vi "PH_gentec_M-Link.Evt Call Set Auto Range.vi"(0 "i ref in":refnum<vi>, 2 "Instance":string, 3 "Set Auto Range":bool, 5 "error in (no error)":errorcluster) -> (14 "i ref out":refnum<vi>, 19 "error out":errorcluster)   [LabVIEW 2014, in "PH_gentec_M-Link.lvlib"]
doc: "This VI calls a certain Proc Event by a simple call."
uses:
  PH_gentec_M-Link.lvlib
  CS_Core/CSSystem/CoreLib/CoreLib.short 2 byte array.vi
  CS_Core/BaseProcess/BaseProcess.lvlib
  CS_Core/CSSystem/CoreLib/CoreLib.lvlib
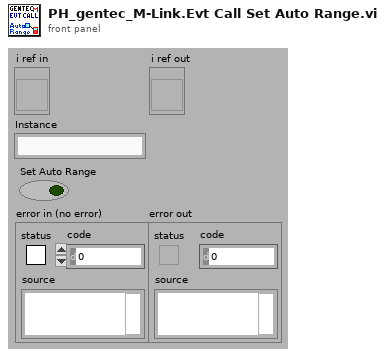
[diagram p1: front panel]
types:
  T1 = typedef "CoreDefs.rawDataType.ctl" = i8[]
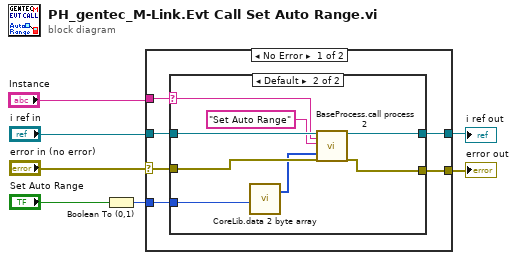
[diagram p0: block diagram]
diagram:
  n1 = Boolean To (0,1)(Boolean="Set Auto Range") -> (0, 1=w1:i16)
  n2 = case shown="No Error" "error in (no error)" {
    selector: "error in (no error)" -> [w8 w24]
    tunnel: [w13 w25] -> w3
    tunnel: [w12 w24] -> w2
    tunnel: "i ref in" -> [w11 w25]
    tunnel: "Instance" -> [w9 _]
    tunnel: w1 -> [w10 _]
    frame No Error {
      n3 = case shown="Default" w9 {
        selector: w9 -> [_ w16]
        tunnel: [w15 w23] -> w13
        tunnel: [w14 w22] -> w12
        tunnel: w11 -> [w15 w21]
        tunnel: w8 -> [w14 w20]
        tunnel: w10 -> [_ w18]
        frame "", "N/A" {
        }
        frame Default {
          n4 = call-poly "CoreLib.data 2 byte array.vi"("i16"=w18) -> ("byteArray out"=w17:T1)  [unwired: 18 in]
          n5 = call "BaseProcess.call process 2.vi"("i ref in"=w21, "Object"=w16, "Selector"="Set Auto Range", "Data"=w17, "error in (no error)"=w20) -> ("i ref out"=w23:refnum<vi>, "error out"=w22:errorcluster)  [unwired: 13 in]
        }
      }
    }
    frame Error {
    }
  }
  "error out" <- w2
  "i ref out" <- w3
